vi "AD7609 sleepmode.vi"(1 "Sleep state":u8(ring) items=["Awake", "Standby", "Shutdown"], 2 "VISA resource name":refnum<visa-resource-name>) -> (0 "Sleep error out":errorcluster)   [LabVIEW 2020]
uses:
  <vilib>/Instr/_visa.llb/VISA Open Access Mode.ctl
panel:
  out "Sleep string output":string
  # "PN 25/11/2014, 17/08/2015"
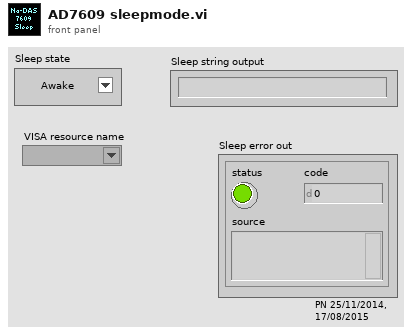
[diagram p1: front panel]
types:
  T1 = typedef "VISA Open Access Mode.ctl" = u32
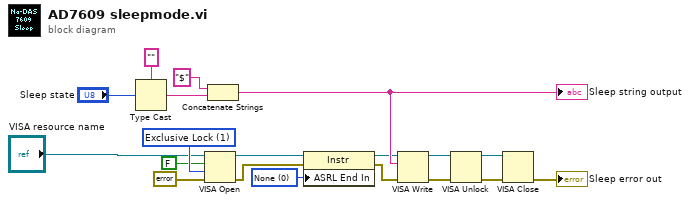
[diagram p0: block diagram]
diagram:
  w6 = u16 0 items=["None", "Last Bit", "TermChar"] ("Serial Settings:End Mode for Reads")
  w15 = T1 1 items=["VISA Defaults"=0, "Exclusive Lock"=1, "Load Configured Settings"=4] ("Access Mode")
  n1 = Type Cast(type="", x="Sleep state") -> (*(type *) &x=w18:string)
  n2 = VISA Open(duplicate session (F)=FALSE, access mode=w15, error in (no error)=errorcluster {"status"=FALSE, "code"=0, "source"=""}, VISA resource name="VISA resource name") -> (VISA resource name=w5:refnum<visa-resource-name>, error out=w4:errorcluster)  [unwired: 1 in]
  n3 = Concatenate Strings("$", w18) -> (w16:string)
  "Sleep string output" <- w16
  n4 = property class="Instr"(reference=w5, error in=w4, "ASRL End In"=w6) -> (reference out=w3:refnum<visa-resource-name>, error out=w2:errorcluster)
  n5 = VISA Write(VISA resource name=w3, write buffer=w16, error in (no error)=w2) -> (VISA resource name out=w10:refnum<visa-resource-name>, error out=w9:errorcluster)  [unwired: 1 out]
  n6 = VISA Unlock(8:w9, 11:w10) -> (0:w12:errorcluster, 3:w13:refnum<visa-resource-name>)
  n7 = VISA Close(VISA resource name=w13, error in (no error)=w12) -> (error out=→"Sleep error out":errorcluster)
